vi "Run.vi"(8 "error in (no error)":errorcluster, 9 "s on last turn":dbl, 10 "Maze (0: Empty, -1: Enemy. >0: Teammate":i32[][](array[numeric]), 11 "Net in":refnum<class "Net.lvclass">) -> (0 "error out":errorcluster, 1 "Direction":T1, 2 "Action":T2, 3 "Net out":refnum<class "Net.lvclass">, 4 "Replicated":refnum<class "Runner.lvclass">)   [LabVIEW 2014, in "Net.lvclass"]
uses:
  Net.lvclass
  Action Enum.ctl
  Direction Enum.ctl
  Runner.lvclass
  Net Attack/Net Attack.lvclass
  SquareBattle.lvclass
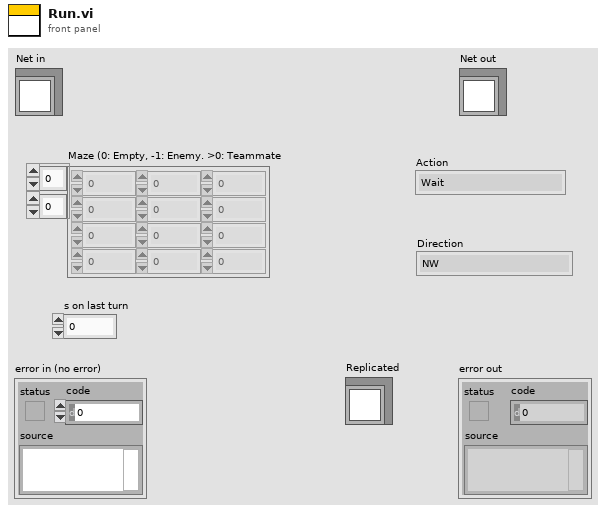
[diagram p1: front panel]
types:
  T1 = typedef "SquareBattle.lvclass/Direction Enum.ctl" = enum16{"NW", "N", "NE", "E", "SE", "S", "SW", "W"}
  T2 = typedef "SquareBattle.lvclass/Action Enum.ctl" = enum16{"Wait", "Move", "Attack", "Replicate"}
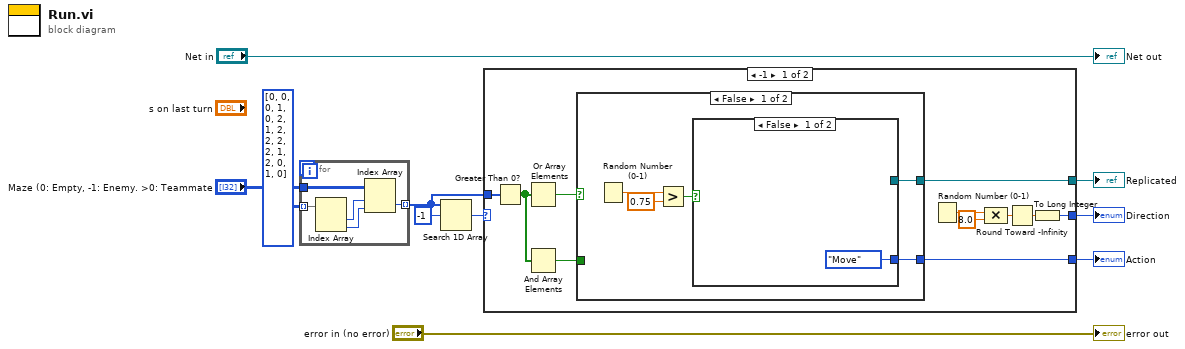
[diagram p0: block diagram]
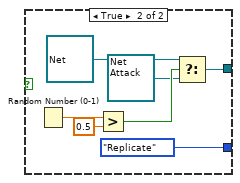
[diagram p2: hidden frame]
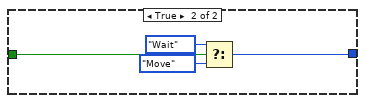
[diagram p3: hidden frame]
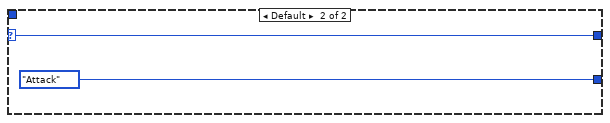
[diagram p4: hidden frame]
diagram:
  n1 = for {
    tunnel: "Maze (0: Empty, -1: Enemy. >0: Teammate" -> [w15]
    tunnel: i32[][] [[0, 0], [0, 1], [0, 2], [1, 2], [2, 2], [2, 1], [2, 0], [1, 0]] -> [w14] mode=indexing
    tunnel: [w11] -> w3 mode=indexing
    n2 = Index Array(array=w14) -> (element #1=w13:i32, element #2=w12:i32)  [unwired: 2 in]
    n3 = Index Array(array=w15, index (row)=w13, index (col)=w12) -> (element=w11:i32)
  }
  n4 = Search 1D Array(1D array=w3, element=-1) -> (index of element=w6:i32)  [unwired: 1 in]
  n5 = case shown="-1" w6 {
    selector: w6 -> [_ w45]
    tunnel: [w21 w45] -> w5
    tunnel: [w18 Action_Enum."Attack" ("Action")] -> w4
    tunnel: w3 -> [w22 _]
    tunnel: [w17 _] -> w2
    frame -1 {
      n6 = Greater Than 0?(x=w22) -> (x > 0?=w20:bool[])
      n7 = Or Array Elements(Boolean array=w20) -> (logical OR=w16:bool)
      n8 = And Array Elements(Boolean array=w20) -> (logical AND=w19:bool)
      n9 = case shown="False" w16 {
        tunnel: w19 -> [_ w43]
        tunnel: [w31 w40] -> w18
        tunnel: [w30 _] -> w17
        frame False {
          n10 = Random Number (0-1)() -> (number: 0 to 1=w29:dbl)
          n11 = Greater?(x=w29, y=0.75) -> (0:w27:bool)
          n12 = case shown="False" w27 {
            tunnel: [Action_Enum."Move" ("f") Action_Enum."Replicate" ("f")] -> w31
            tunnel: [_ w34] -> w30
            frame False {
            }
            frame True {
              n13 = Random Number (0-1)() -> (number: 0 to 1=w38:dbl)
              n14 = Greater?(x=w38, y=0.5) -> (0:w36:bool)
              n15 = Select(t=refnum<class "Net.lvclass"> refnum ("Net.lvclass"), s=w36, f=refnum<class "Net Attack.lvclass"> refnum ("Net Attack.lvclass")) -> (s? t:f=w34:refnum<class "Runner.lvclass">)
            }
          }
        }
        frame True {
          n16 = Select(t=Action_Enum."Wait" ("Action"), s=w43, f=Action_Enum."Move") -> (s? t:f=w40:T2)
        }
      }
      n17 = Random Number (0-1)() -> (number: 0 to 1=w26:dbl)
      n18 = Compound Arithmetic op=MULTIPLY(w26, 8.0 ("value")) -> (w24:dbl)
      n19 = Round Toward -Infinity(1:w24) -> (0:w23:dbl)
      n20 = To Long Integer(number=w23) -> (32bit integer=w21:i32)
    }
    frame Default {
    }
  }
  "Action" <- w4
  "Direction" <- w5
  "Replicated" <- w2
  "error out" <- "error in (no error)"
  "Net out" <- "Net in"
